vi "Commit Transaction.vi"(8 "error in (no error)":errorcluster, 11 "Sqlite Database Manager in":refnum<class "Sqlite Database Manager.lvclass">) -> (0 "error out":errorcluster, 3 "Sqlite Database Manager out":refnum<class "Sqlite Database Manager.lvclass">)   [LabVIEW 2019, in "HierDAL Library.lvlib" / "Database.lvlib" / "Sqlite Database Manager.lvclass"]
uses:
  Sqlite Database Manager.lvclass
  Sqlite Database Manager.lvclass/Sqlite Database Manager.ctl
  System.Data.SQLite
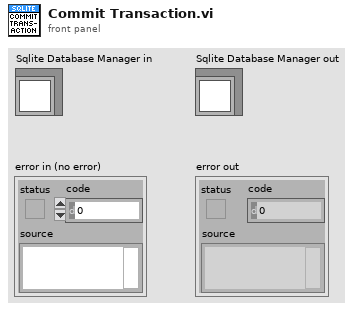
[diagram p1: front panel]
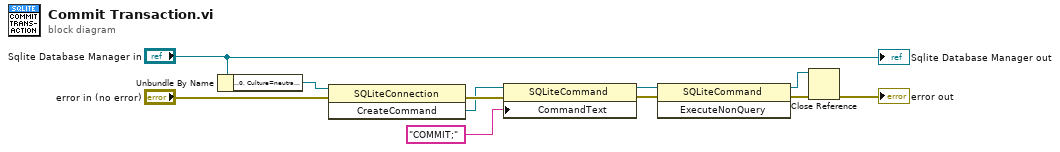
[diagram p0: block diagram]
diagram:
  n1 = Unbundle By Name("Sqlite Database Manager in") -> ("Connection"=w11:refnum<k24>)
  n2 = invoke class="SQLiteConnection" method="CreateCommand"(reference=w11, error in="error in (no error)") -> (error out=w10:errorcluster, "CreateCommand"=w9:refnum<k24>)  [unwired: 1 in, 1 out]
  n3 = property class="SQLiteCommand"(reference=w9, error in=w10, "CommandText"="COMMIT;") -> (reference out=w6:refnum<k24>, error out=w7:errorcluster)
  n4 = invoke class="SQLiteCommand" method="ExecuteNonQuery"(reference=w6, error in=w7) -> (reference out=w4:refnum<k24>, error out=w5:errorcluster)  [unwired: 1 in, 1 out]
  n5 = Close Reference(reference=w4, error in (no error)=w5) -> (error out=→"error out":errorcluster)
  "Sqlite Database Manager out" <- "Sqlite Database Manager in"
